vi "145.vi"() -> ()   [LabVIEW 2021]
panel:
  out "size(s)":i32
  in  "Limit":i32
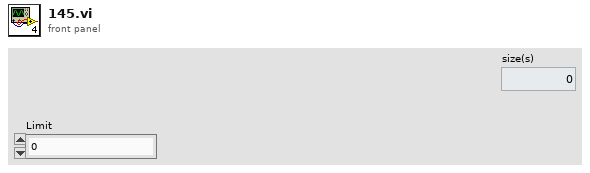
[diagram p1: front panel]
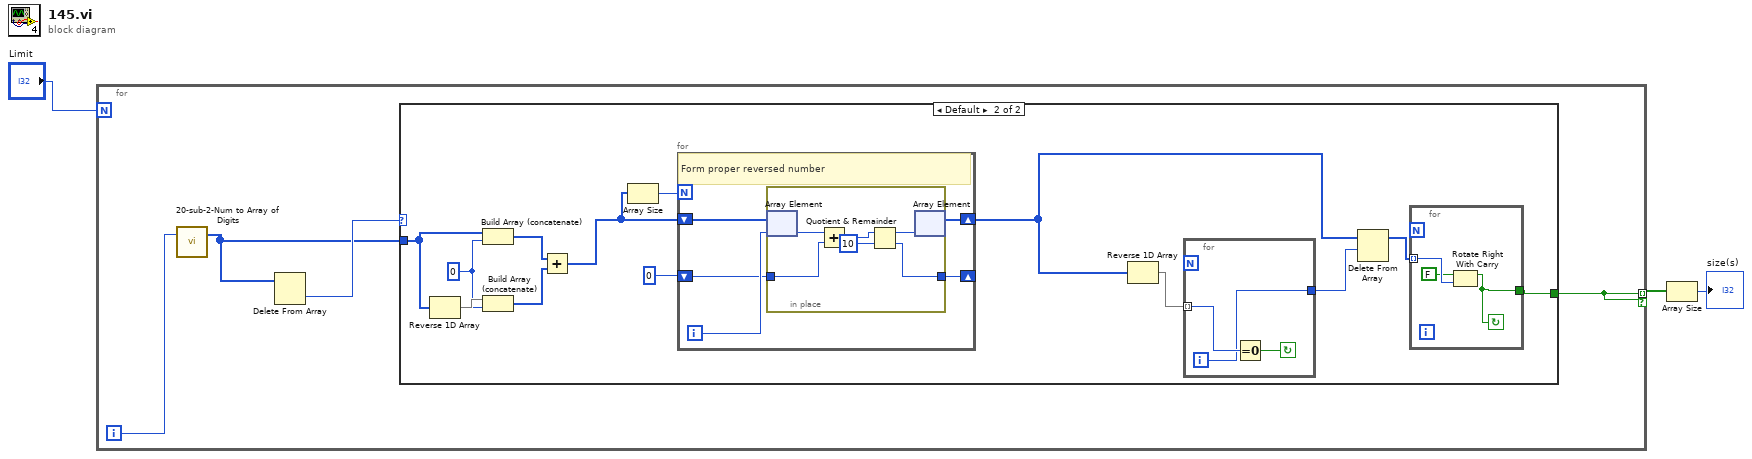
[diagram p0: block diagram]
diagram:
  n1 = for {
    N: "Limit" -> [_]
    tunnel: [w4] -> w2 mode=indexing if=w4
    i -> [w7]
    n2 = call "20-sub-2-Num to Array of Digits.vi"("N"=w7) -> ("N as Array"=w5:u8[])  [unwired: 2 in]
    n3 = Delete From Array(array=w5) -> (deleted portion=w6:u8)  [unwired: 2 in, 1 out]
    n4 = case shown="Default" w6 {
      tunnel: w5 -> [_ w20]
      tunnel: [_ w8] -> w4
      frame 0 {
        # "Ends in zero. So reverse will have leading zero"
      }
      frame Default {
        w18 = u8 0 ("element")
        n5 = Reverse 1D Array(array=w20) -> (reversed array=w19:u8[])
        n6 = Build Array (concatenate)(w20, w18) -> (w17:u8[])
        n7 = Build Array (concatenate)(w19, w18) -> (w16:u8[])
        n8 = Add(x=w17, y=w16) -> (x+y=w13:u8[])
        n9 = Array Size(array=w13) -> (size(s)=w15:i32)
        n10 = for {
          N: w15 -> [_]
          shift-right: [w30] -> w10
          shift-left: w13 -> [w31]
          shift-right: [w27] -> _
          shift-left: u8 0 -> [w28]
          i -> [w29]
          # "Form proper reversed number"
          n11 = in-place {
            in-place-border: w28 -> [w33]
            in-place-border: [w32] -> w27
            n12 = in-place-array #1(w31, w29) -> (w37:u8)
            n13 = Add(x=w37, y=w33) -> (x+y=w34:u8)
            n14 = Quotient & Remainder(x=w34, y=u8 10) -> (x-y*floor(x/y)=w35:u8, floor(x/y)=w32:u8)
            n15 = in-place-array #1(w35) -> (w30:u8[])  [unwired: 1 out]
          }
        }
        n16 = Reverse 1D Array(array=w10) -> (reversed array=w12:u8[])
        n17 = for {
          tunnel: w12 -> [w26] mode=indexing
          tunnel: [w24] -> w11
          i -> [w24]
          stop <- w25 continue-if-true
          n18 = Equal To 0?(x=w26) -> (x = 0?=w25:bool)
        }
        n19 = Delete From Array(array=w10, length=w11) -> (array with subset deleted=w9:u8[])  [unwired: 1 in, 1 out]
        n20 = for {
          tunnel: w9 -> [w23] mode=indexing
          tunnel: [w21] -> w8
          stop <- w21 continue-if-true
          n21 = Rotate Right With Carry(2:w23, 3:FALSE ("carry")) -> (1:w21:bool)  [unwired: 1 out]
        }
      }
    }
  }
  n22 = Array Size(array=w2) -> (size(s)=→"size(s)":i32)
